vi "LMS_Close.vi"(8 "error in (no error)":errorcluster, 11 "device_In":i64) -> (0 "error out":errorcluster)   [LabVIEW 2018, in "LMS_LV_Drv.lvlib"]
uses:
  LMS_LV_Drv.lvlib
  C:/Program Files/PothosSDR/bin/LimeSuite.dll
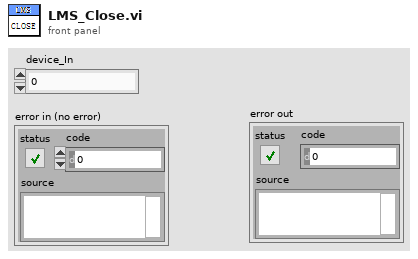
[diagram p1: front panel]
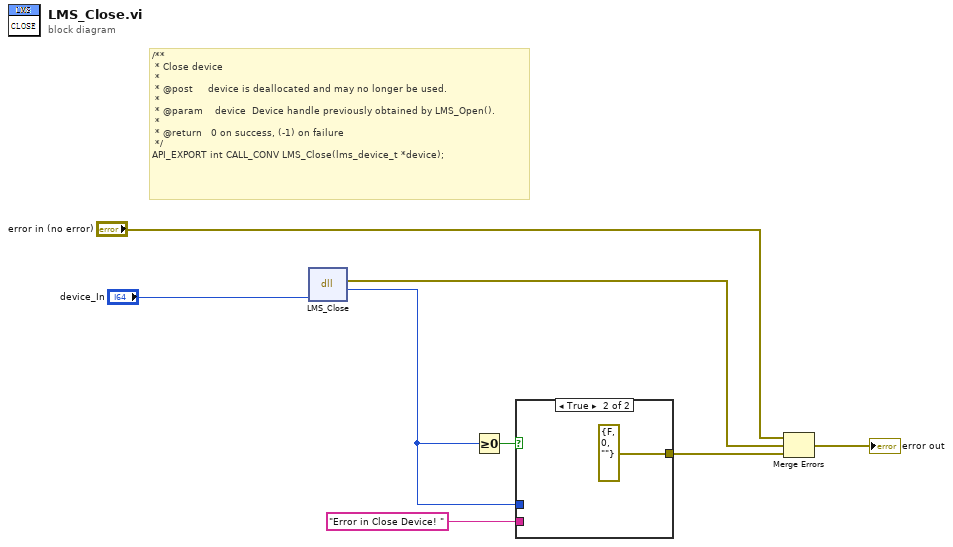
[diagram p0: block diagram]
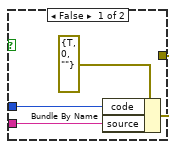
[diagram p2: hidden frame]
diagram:
  # "/**\n * Close device\n *\n * @post     device is deallocated and may no longer be used.\n *\n * @param    device  Device handle previously obtained by LMS_Open().\n *\n * @return   0 on success, (-1) on failure\n */\nAPI_EXPORT int CALL_CONV LMS_Close(lms_device_t *device);"
  n1 = dll-call lib="C:/Program Files/PothosSDR/bin/LimeSuite.dll" fn="LMS_Close"("device"="device_In") -> (error out=w3:errorcluster, "return type"=w4:i32)  [unwired: 4 in, 1 out]
  n2 = Greater Or Equal To 0?(x=w4) -> (x >= 0?=w7:bool)
  n3 = case shown="True" w7 {
    tunnel: [w11 errorcluster {"status"=FALSE, "code"=0, "source"=""} ("error in")] -> w5
    tunnel: w4 -> [w10 _]
    tunnel: "Error in Close Device! " ("source") -> [w9 _]
    frame False {
      n4 = Bundle By Name(cluster=errorcluster {"status"=TRUE, "code"=0, "source"=""} ("error in"), "code"=w10, "source"=w9) -> (w11:errorcluster)
    }
    frame True {
    }
  }
  n5 = Merge Errors("error in (no error)", w3, w5) -> (→"error out":errorcluster)
